vi "Respondedor.vi"() -> ()   [LabVIEW 2018]
uses:
  RxTx/RxTx.lvclass
panel:
  out "error out 2":errorcluster
  in  "Queue RX":refnum<class "RxTx.lvclass">
  out "Received request":string
  in  "stop":bool
  # "REP endpoint"
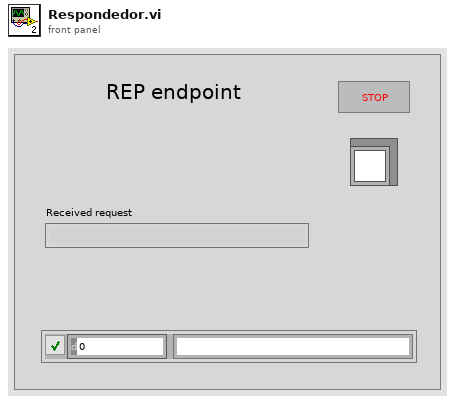
[diagram p1: front panel]
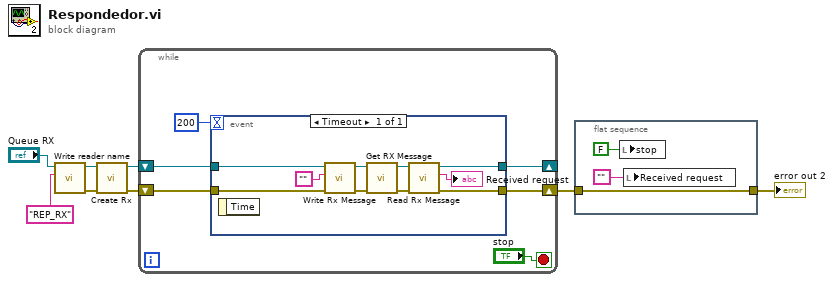
[diagram p0: block diagram]
diagram:
  n1 = call-dynamic "Write reader name.vi"("RX name"="REP_RX", "RxTx in"="Queue RX") -> ("error out"=w5:errorcluster, "RxTx out"=w6:refnum<class "RxTx.lvclass">)  [unwired: 8 in]
  n2 = call "Create Rx.vi"("error in (no error)"=w5, "RxTx in"=w6) -> ("error out"=w4:errorcluster, "RxTx out"=w8:refnum<class "RxTx.lvclass">)  [unwired: 8 in]
  n3 = while {
    shift-right: [w11] -> _
    shift-left: w8 -> [w13]
    shift-right: [w10] -> w3
    shift-left: w4 -> [w12]
    stop <- "stop" stop-if-true
    n4 = event shown="[0] Timeout" {
      selector: _ -> [_]
      dyn-events: _ -> [_]
      timeout: 200 -> [_]
      tunnel: [w21] -> w11
      tunnel: [w18] -> w10
      tunnel: w13 -> [w16]
      tunnel: w12 -> [w15]
      event Timeout {
        n5 = event-data() -> ()  [unwired: 1 in, 1 out]
        n6 = call "Write Rx Message.vi"("error in (no error)"=w15, "Rx Message"="", "RxTx in"=w16) -> ("error out"=w20:errorcluster, "RxTx out"=w22:refnum<class "RxTx.lvclass">)  [unwired: 7 in]
        n7 = call "Get RX Message.vi"("error in (no error)"=w20, "RxTx in"=w22) -> ("error out"=w23:errorcluster, "RxTx out"=w24:refnum<class "RxTx.lvclass">)  [unwired: 7 in, 1 out]
        n8 = call "Read Rx Message.vi"("error in (no error)"=w23, "RxTx in"=w24) -> ("error out"=w18:errorcluster, "Rx Message"=→"Received request":string, "RxTx out"=w21:refnum<class "RxTx.lvclass">)  [unwired: 7 in]
      }
    }
  }
  n9 = flat-sequence {
    tunnel: w3 -> [w27]
    tunnel: [w27] -> w2
    frame #0 {
      n10 = local write "stop"(FALSE ("stop")) -> ()
      n11 = local write "Received request"("") -> ()
    }
  }
  "error out 2" <- w2
